vi "Write Output.vi"(8 "error in (no error)":errorcluster, 11 "Bioreactor in":refnum<class "Bioreactor.lvclass">) -> (0 "error out":errorcluster, 3 "Bioreactor out":refnum<class "Bioreactor.lvclass">)   [LabVIEW 2012]
uses:
  Bioreactor.lvclass
  Bioreactor.lvclass/Bioreactor.ctl
  Read Address.vi
  Read VISA resource name.vi
  Read DVR.vi
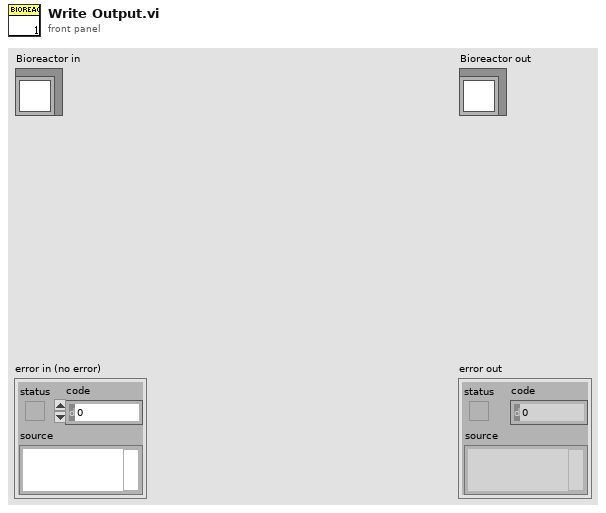
[diagram p1: front panel]
types:
  T1 = cluster{"Name":string, "Value":dbl, "Setpoint":dbl, "Output":dbl}[]
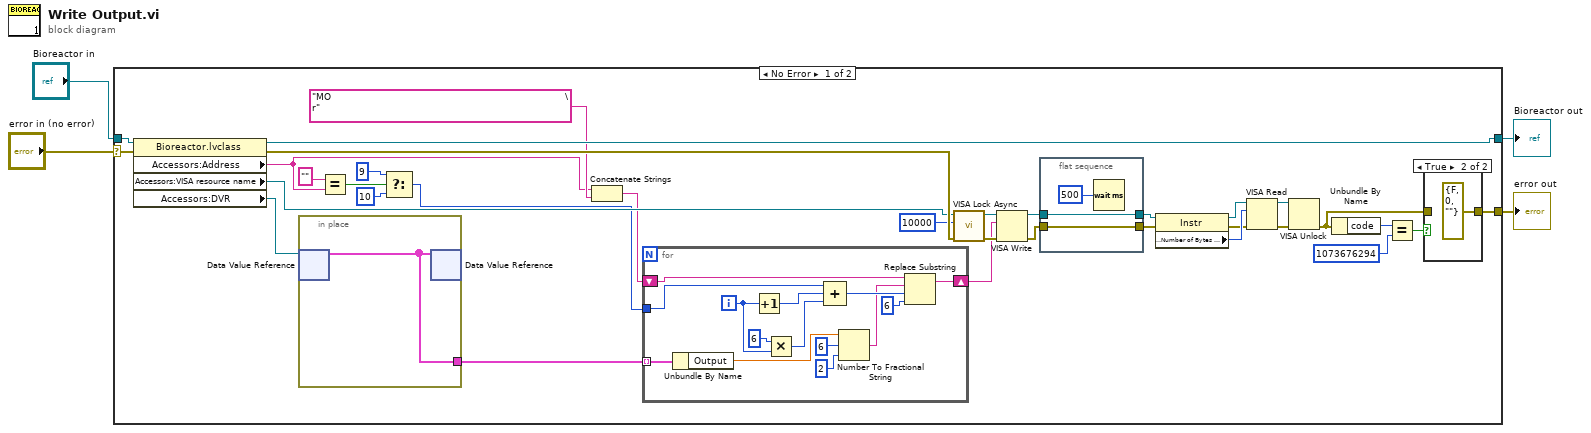
[diagram p0: block diagram]
diagram:
  n1 = case shown="No Error" "error in (no error)" {
    selector: "error in (no error)" -> [w27 w59]
    tunnel: [w17 w59] -> w1
    tunnel: [w16 w58] -> w2
    tunnel: "Bioreactor in" -> [w26 w58]
    frame No Error {
      n2 = property class="Bioreactor.lvclass"(reference=w26, error in=w27) -> (reference out=w16:refnum<class "Bioreactor.lvclass">, error out=w25:errorcluster, "Accessors:Address"=w5:string, "Accessors:VISA resource name"=w14:refnum<visa-resource-name>, "Accessors:DVR"=w18:refnum<data-value>)
      n3 = in-place {
        in-place-border: [w52] -> w15
        n4 = in-place-dvr #1(w18) -> (w52:T1)  [unwired: 1 out]
        n5 = in-place-dvr #1(w52) -> ()  [unwired: 2 out]
      }
      n6 = Equal?(x="", y=w5) -> (x = y?=w10:bool)
      n7 = Select(t=9, s=w10, f=10) -> (s? t:f=w6:i32)
      n8 = Concatenate Strings(w5, "MO                                                                              \r" ("y")) -> (w12:string)
      n9 = for {
        tunnel: w6 -> [w51]
        tunnel: w15 -> [w44] mode=indexing
        shift-right: [w42] -> w11
        shift-left: w12 -> [w43]
        i -> [w47]
        n10 = Unbundle By Name(w44) -> ("Output"=w39:dbl)
        n11 = Increment(x=w47) -> (x+1=w49:i32)
        n12 = Multiply(x=6, y=w47) -> (x*y=w46:i32)
        n13 = Compound Arithmetic op=ADD(w51, w49, w46) -> (w50:i32)
        n14 = Number To Fractional String(number=w39, width (-)=i16 6, precision (6)=i16 2 ("width (-)")) -> (F-format string=w38:string)  [unwired: 1 in]
        n15 = Replace Substring(2:6, 3:w50, 4:w38, 5:w43) -> (1:w42:string)  [unwired: 1 out]
      }
      n16 = call <vilib>:"VISA Lock Async.vi"("error in (no error)"=w25, "timeout (0)"=u32 10000, "VISA resource name"=w14) -> ("error out"=w24:errorcluster, "VISA resource name out"=w23:refnum<visa-resource-name>)  [unwired: 6 in, 1 out]
      n17 = VISA Write(VISA resource name=w23, write buffer=w11, error in (no error)=w24) -> (VISA resource name out=w34:refnum<visa-resource-name>, error out=w32:errorcluster)  [unwired: 1 out]
      n18 = flat-sequence {
        tunnel: [w57] -> w33
        tunnel: w34 -> [w57]
        tunnel: [w56] -> w31
        tunnel: w32 -> [w56]
        frame #0 {
          n19 = Wait (ms)(milliseconds to wait=500 ("y")) -> ()  [unwired: 1 out]
        }
      }
      n20 = property class="Instr"(reference=w33, error in=w31) -> (reference out=w35:refnum<visa-resource-name>, error out=w36:errorcluster, "Serial Settings:Number of Bytes at Serial Port"=w37:u32)
      n21 = VISA Read(VISA resource name=w35, byte count=w37, error in (no error)=w36) -> (VISA resource name out=w19:refnum<visa-resource-name>, error out=w21:errorcluster)  [unwired: 2 out]
      n22 = VISA Unlock(8:w21, 11:w19) -> (0:w20:errorcluster)  [unwired: 1 out]
      n23 = Unbundle By Name(w20) -> ("code"=w30:i32)
      n24 = Equal?(x=w30, y=1073676294) -> (x = y?=w28:bool)
      n25 = case shown="True" w28 {
        tunnel: w20 -> [w53 _]
        tunnel: [w53 errorcluster {"status"=FALSE, "code"=0, "source"=""} ("error constant")] -> w17
        frame False {
        }
        frame True {
        }
      }
    }
    frame Error {
    }
  }
  "error out" <- w1
  "Bioreactor out" <- w2
